vi "Device Discovery Tester.vi"() -> ()   [LabVIEW 2016]
uses:
  <vilib>/ORNL/CSEISMIC DDS/CSEISMIC DDS Base/CSEISMIC DDS.lvclass/CSEISMIC DDS.ctl
  <vilib>/ORNL/CSEISMIC DDS/CSEISMIC DDS Base/Accessors/Write DDS Reference.vi
  <vilib>/ORNL/CSEISMIC DDS/CSEISMIC DDS Base/Accessors/Read DDS Reference.vi
  <vilib>/ORNL/CSEISMIC DDS/DDS Reader/DDS Reader.lvclass
  C:/Program Files (x86)/National Instruments/LabVIEW 2016/vi.lib/ORNL/CSEISMIC DDS/CSEISMIC DDS Base/CSEISMIC DDS.lvclass
  <vilib>/ORNL/CSEISMIC DDS/CSEISMIC DDS Base/Error Handler.vi
panel:
  out "error out":errorcluster
  in  "stop":bool
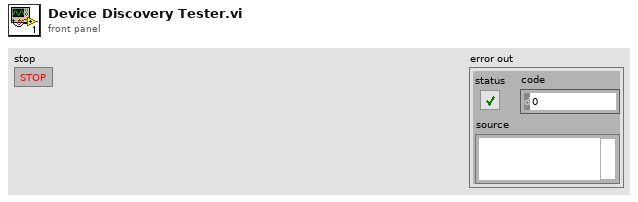
[diagram p1: front panel]
types:
  T1 = enum16{"open", "open or create", "create or replace", "create", "open (read-only)"}
  T2 = typedef "CSEISMIC DDS.lvlib/CSEISMIC DDS.lvclass/IED_Status.ctl" = cluster{"DeviceID":T3, "Timestamp":T4, "MicrogridID":u8, "Active":bool, "Inactive":bool, "Error":i32, "Fault":bool, "ErrorString":string}
  T3 = typedef "CSEISMIC DDS.lvlib/CSEISMIC DDS.lvclass/DeviceID.ctl" = string
  T4 = typedef "CSEISMIC DDS.lvlib/CSEISMIC DDS.lvclass/Timestamp.ctl" = cluster{"Seconds":u64, "Remainder":u64}
  T5 = typedef "LVDDS_library.lvlib/DDS Sample Info.ctl" = cluster{"DDS_SampleStateKind":enum32{"DDS_INVALID_SAMPLE_STATE", "DDS_READ_SAMPLE_STATE", "DDS_NOT_READ_SAMPLE_STATE"}, "DDS_ViewStateKind":enum32{"DDS_INVALID_SAMPLE_STATE", "DDS_NEW_VIEW_STATE", "DDS_NOT_NEW_VIEW_STATE"}, "DDS_InstanceStateKind":enum32{"DDS_INVALID_STATE", "DDS_ALIVE_INSTANCE_STATE", "DDS_NOT_ALIVE_DISPOSED_INSTANCE_STATE", "", "DDS_NOT_ALIVE_NO_WRITERS_INSTANCE_STATE"}, "sec":i32, "nanosec":u32, "valid_data":bool}
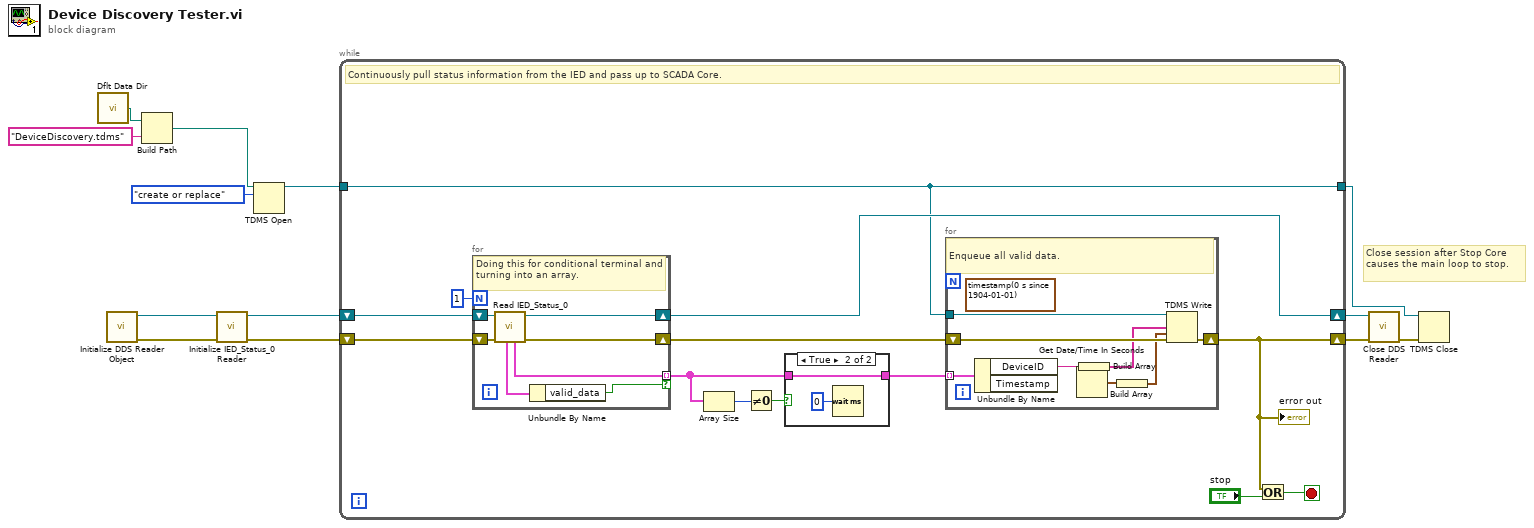
[diagram p0: block diagram]
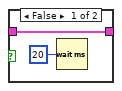
[diagram p2: hidden frame]
diagram:
  # "Close session after Stop Core causes the main loop to stop."
  n1 = call <vilib>:"Dflt Data Dir.vi"() -> ("App:Default Data Directory"=w7:path)
  n2 = call <vilib>:"Initialize DDS Reader Object.vi"() -> ("error out"=w12:errorcluster, "DDS Reader out"=w13:refnum<class "DDS Reader.lvclass">)  [unwired: 10 in]
  n3 = Build Path(base path=w7, name or relative path="DeviceDiscovery.tdms") -> (appended path=w5:path)
  n4 = call <vilib>:"Initialize IED_Status_0 Reader.vi"("error in"=w12, "DDS Reader in"=w13) -> ("error out"=w10:errorcluster, "DDS Reader out"=w11:refnum<class "DDS Reader.lvclass">)  [unwired: 8 in]
  n5 = TDMS Open(10:T1."create or replace" ("operation (0:open)"), 11:w5) -> (3:w3:refnum<k34>)  [unwired: 5 in, 1 out]
  n6 = while {
    shift-right: [w14] -> w8
    shift-left: w10 -> [w25]
    shift-right: [w24] -> w9
    shift-left: w11 -> [w26]
    tunnel: w3 -> [w17]
    tunnel: [w17] -> w1
    stop <- w16 stop-if-true
    # "Continuously pull status information from the IED and pass up to SCADA Core."
    n7 = for {
      N: 1 -> [_]
      shift-right: [w43] -> w24
      shift-left: w26 -> [w45]
      shift-right: [w42] -> w22
      shift-left: w25 -> [w44]
      tunnel: [w40] -> w19 mode=indexing if=w39
      # "Doing this for conditional terminal and turning into an array."
      n8 = call <vilib>:"Read IED_Status_0.vi"("error in"=w44, "DDS Reader in"=w45) -> ("error out"=w42:errorcluster, "DDS Reader out"=w43:refnum<class "DDS Reader.lvclass">, "data"=w40:T2, "DDS Sample Info"=w41:T5)  [unwired: 6 in]
      n9 = Unbundle By Name(w41) -> ("valid_data"=w39:bool)
    }
    n10 = Array Size(array=w19) -> (size(s)=w21:i32)
    n11 = Not Equal To 0?(x=w21) -> (x != 0?=w20:bool)
    n12 = case shown="True" w20 {
      tunnel: w19 -> [w28 w29]
      tunnel: [w28 w29] -> w18
      frame False {
        n13 = Wait (ms)(milliseconds to wait=u32 20) -> ()  [unwired: 1 out]
      }
      frame True {
        n14 = Wait (ms)(milliseconds to wait=u32 0) -> ()  [unwired: 1 out]
      }
    }
    n15 = for {
      tunnel: w18 -> [w36] mode=indexing
      shift-right: [w32] -> w14
      shift-left: w22 -> [w38]
      tunnel: w17 -> [w37]
      (unwired) timestamp(0 s since 1904-01-01)
      # "Enqueue all valid data."
      n16 = Unbundle By Name(w36) -> ("DeviceID"=w35:T3)  [unwired: 1 out]
      n17 = Get Date/Time In Seconds() -> (seconds since 1Jan1904=w31:timestamp)
      n18 = Build Array(w35) -> (w33:T3[])
      n19 = Build Array(w31) -> (w34:timestamp[])
      n20 = TDMS Write(0:w37, 7:w33, 9:w34, 11:w38) -> (15:w32:errorcluster)  [unwired: 2 in, 3 out]
    }
    "error out" <- w14
    n21 = Or(x=w14, y="stop") -> (x .or. y?=w16:bool)
  }
  n22 = call <vilib>:"Close DDS Reader.vi"("error in"=w8, "DDS Reader in"=w9) -> ("error out"=w2:errorcluster)  [unwired: 9 in]
  n23 = TDMS Close(8:w2, 11:w1) -> ()  [unwired: 2 out]
